vi "Compare.vi"(8 "error in (no error)":errorcluster, 10 "Level":dbl, 11 "Percent Difference in":refnum<class "Percent Difference.lvclass">) -> (0 "error out":errorcluster, 2 "Color":u32(colorbox))   [LabVIEW 2021, in "Percent Difference.lvclass"]
uses:
  Percent Difference.lvclass
  Utilities/Colors.ctl
  Percent Difference.lvclass/Percent Difference.ctl
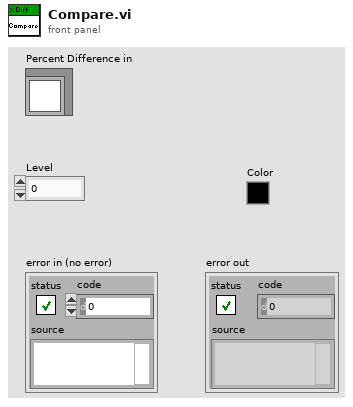
[diagram p1: front panel]
types:
  T1 = typedef "Colors.ctl" = cluster{"Green":u32, "Yellow":u32, "Red":u32}
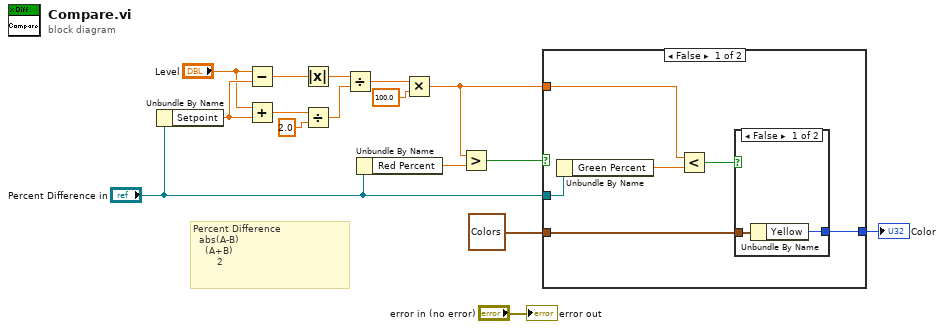
[diagram p0: block diagram]
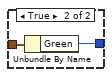
[diagram p2: hidden frame]
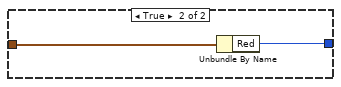
[diagram p3: hidden frame]
diagram:
  # "Percent Difference\n  abs(A-B)\n    (A+B)\n        2"
  n1 = Unbundle By Name("Percent Difference in") -> ("Setpoint"=w2:dbl)
  n2 = Subtract(x="Level", y=w2) -> (x-y=w15:dbl)
  n3 = Add(x="Level", y=w2) -> (x+y=w13:dbl)
  n4 = Absolute Value(x=w15) -> (abs(x)=w14:dbl)
  n5 = Divide(x=w13, y=2.0) -> (x/y=w11:dbl)
  n6 = Divide(x=w14, y=w11) -> (x/y=w9:dbl)
  n7 = Unbundle By Name("Percent Difference in") -> ("Red Percent"=w5:dbl)
  n8 = Multiply(x=w9, y=100.0) -> (x*y=w7:dbl)
  n9 = Greater?(x=w7, y=w5) -> (0:w8:bool)
  n10 = case shown="False" w8 {
    tunnel: [w22 w27] -> w6
    tunnel: w7 -> [w20 _]
    tunnel: T1 {"Green"=65408, "Yellow"=16777088, "Red"=16744576} ("Colors") -> [w17 w28]
    tunnel: "Percent Difference in" -> [w19 _]
    frame False {
      n11 = Unbundle By Name(w19) -> ("Green Percent"=w18:dbl)
      n12 = Less?(x=w20, y=w18) -> (x < y?=w21:bool)
      n13 = case shown="False" w21 {
        tunnel: [w23 w25] -> w22
        tunnel: w17 -> [w24 w26]
        frame False {
          n14 = Unbundle By Name(w24) -> ("Yellow"=w23:u32)
        }
        frame True {
          n15 = Unbundle By Name(w26) -> ("Green"=w25:u32)
        }
      }
    }
    frame True {
      n16 = Unbundle By Name(w28) -> ("Red"=w27:u32)
    }
  }
  "Color" <- w6
  "error out" <- "error in (no error)"
